vi "Database Driver Report Analysis.vi"(4 "Create Table":T4={"table"="", "column information"=[], "primary key (-1)"=-1, "use file? (F)"=FALSE}, 5 "Insert Data":T1, 6 "Options":T6=enum."Select Data", 7 "SQLTableData":T5, 8 "error in":errorcluster, 9 "SQL query":string, 10 "Select":enum16{"SelectWithQuery", "SelectWithColumn"}(ring), 11 "table":string) -> (0 "error out":errorcluster, 1 "tables":string[](array[string]), 2 "Database out":refnum<class "Database.lvclass">, 3 "data":string[][](array[string]))   [LabVIEW 2023, in "HardwareAbstractionLayer_LVOOP.lvlib" / "Database.lvclass"]
doc: "This VI used to Database action engine.\n\n// Defeault Case Select Query"
uses:
  Database.lvclass
  Control/DB Options.ctl
  <vilib>/addons/database/Auxilliary.llb/DB Tools Column Info.ctl
  <vilib>/addons/database/Auxilliary.llb/DB Tools DataTypes.ctl
  Control/DB Selection.ctl
  MYSQL Database_class/MYSQL Database.lvclass
  SQLite Database_class/SQLite Database.lvclass
  Database.lvclass/Database.ctl
  D:/eDCU LTT/VT LTT Project/Source Code/HardwareAbstractionLayer_LVOOP/Database/Database.lvclass
  D:/eDCU LTT/VT LTT Project/Source Code/HardwareAbstractionLayer_LVOOP/Database/MYSQL Database_class/MYSQL Database.lvclass
  D:/eDCU LTT/VT LTT Project/Source Code/HardwareAbstractionLayer_LVOOP/Database/SQLite Database_class/SQLite Database.lvclass
  <vilib>/addons/database/NI_Database_API.lvlib
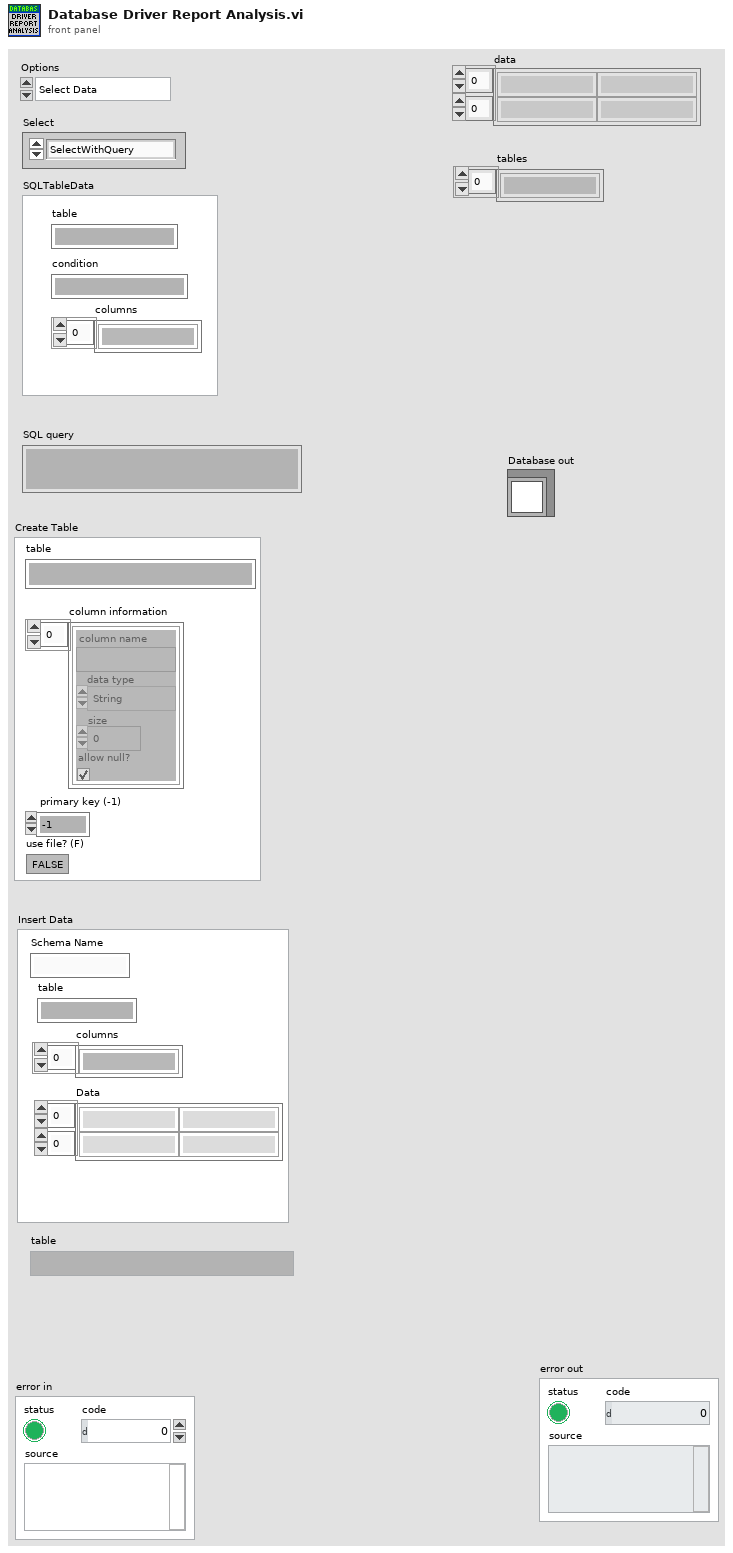
[diagram p1: front panel]
types:
  T1 = cluster{"table":string, "columns":string[], "Data":string[][], "Schema Name":string}
  T2 = typedef "NI_Database_API.lvlib/DB Tools Column Info.ctl" = cluster{"column name":string, "data type":T3, "size":i32, "allow null?":bool}
  T3 = typedef "NI_Database_API.lvlib/DB Tools DataTypes.ctl" = enum16{"String", "Long (I32)", "Single (SGL)", "Double (DBL)", "Date/Time", "Binary"}
  T4 = cluster{"table":string, "column information":T2[], "primary key (-1)":i32, "use file? (F)":bool}
  T5 = cluster{"table":string, "condition":string, "columns":string[]}
  T6 = typedef "HardwareAbstractionLayer_LVOOP.lvlib/Database.lvclass/DB Options.ctl" = enum16{"Init", "Select Data", "Insert Data", "Update Data", "Delete Data", "Execute Query", "Create Schema", "Create Table", "List Tables", "List Columns", "Close"}
  T7 = cluster{"DataSource Name":string, "userID":string, "password":string}
  T8 = enum16{"open", "replace", "create", "open or create", "replace or create", "replace or create with confirmation"}
  T9 = typedef "HardwareAbstractionLayer_LVOOP.lvlib/Database.lvclass/DB Selection.ctl" = string
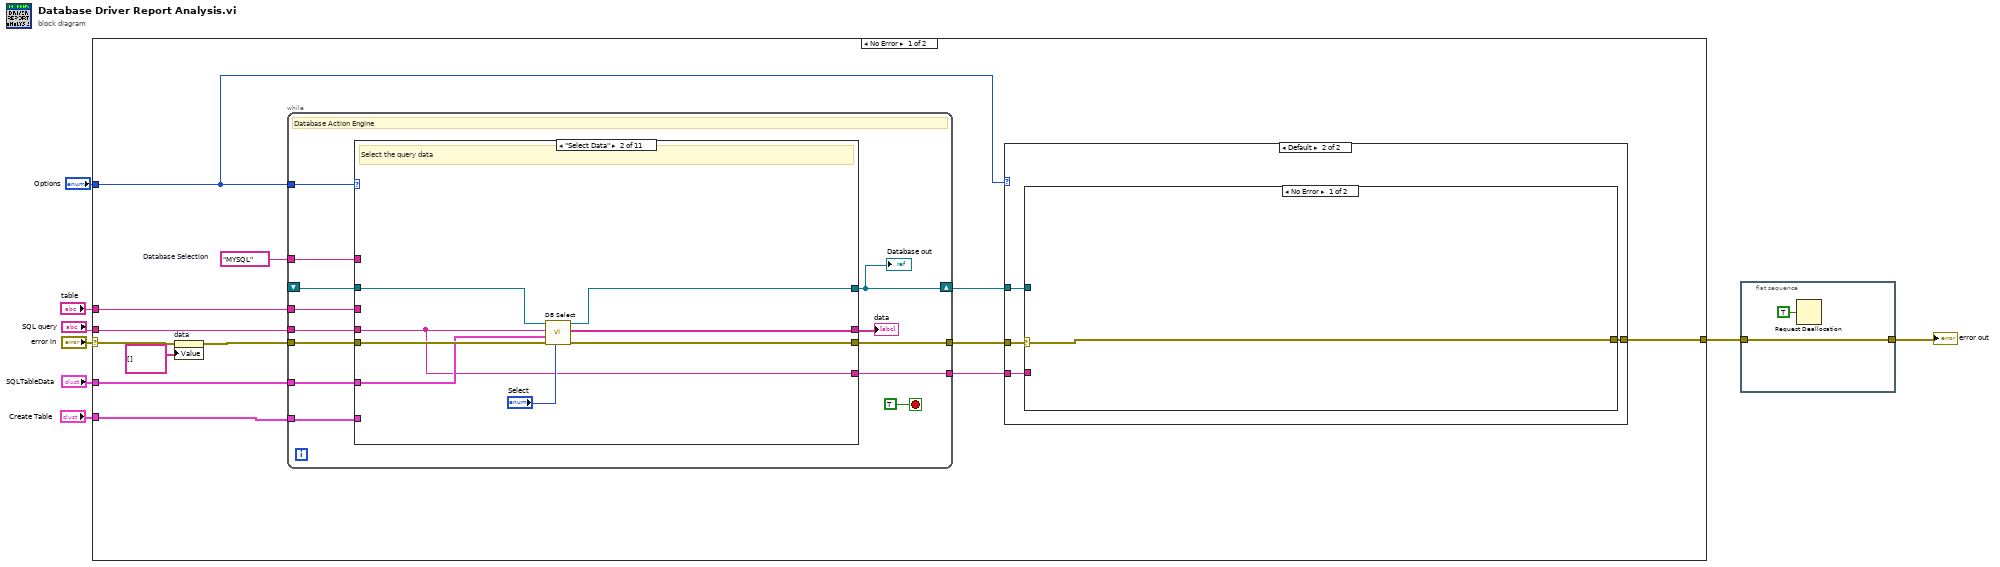
[diagram p0: block diagram]
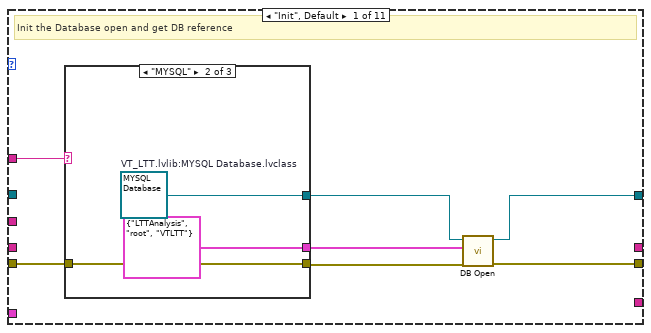
[diagram p2: hidden frame]
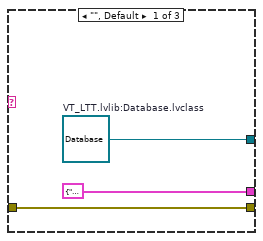
[diagram p3: hidden frame]
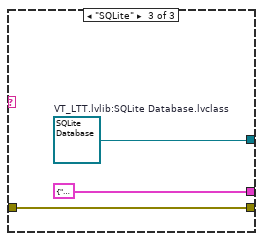
[diagram p4: hidden frame]
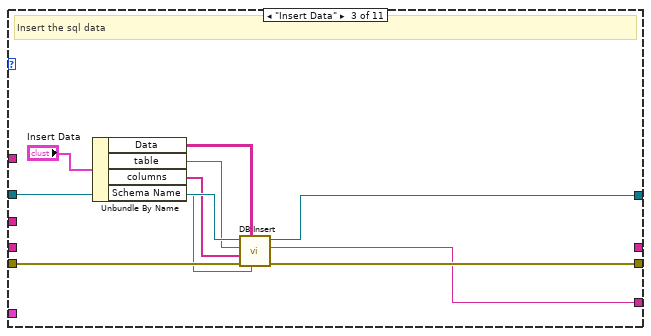
[diagram p5: hidden frame]
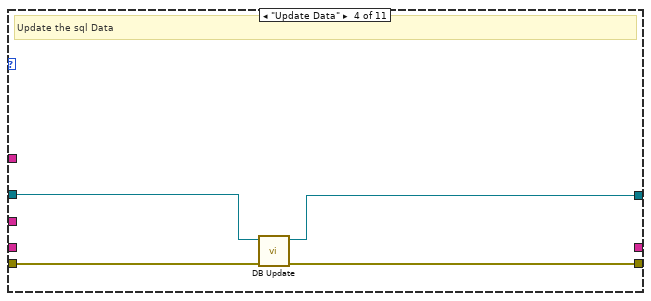
[diagram p6: hidden frame]
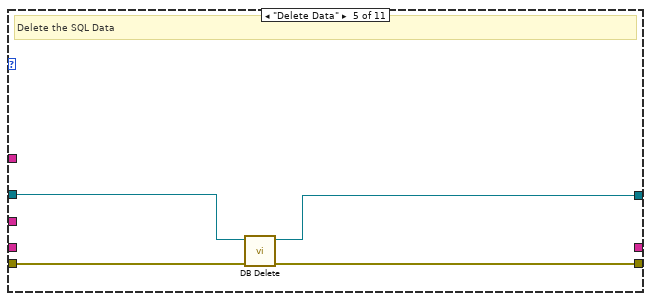
[diagram p7: hidden frame]
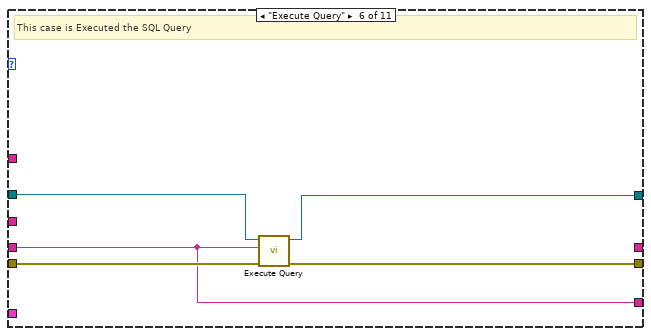
[diagram p8: hidden frame]
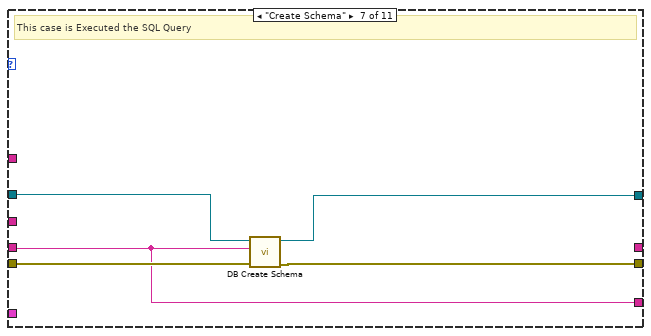
[diagram p9: hidden frame]
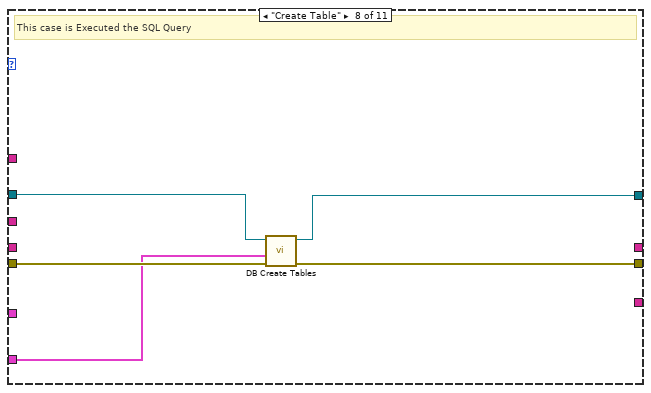
[diagram p10: hidden frame]
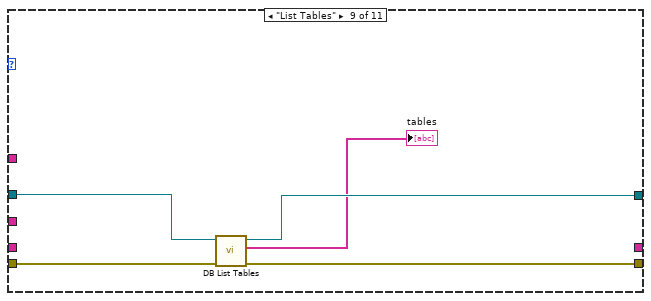
[diagram p11: hidden frame]
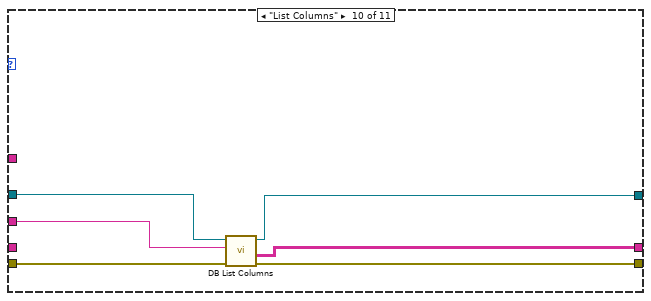
[diagram p12: hidden frame]
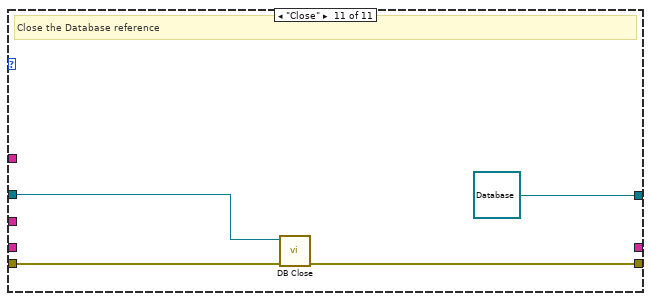
[diagram p13: hidden frame]
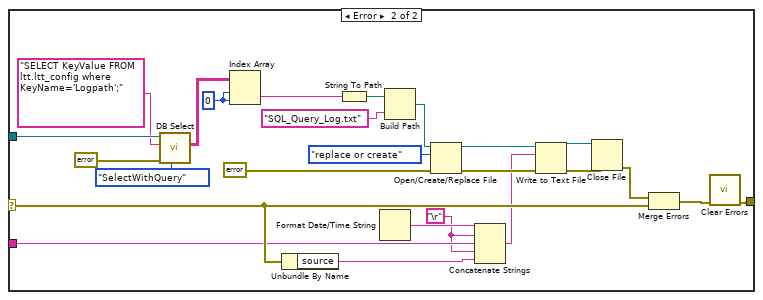
[diagram p15: hidden frame]
diagram:
  n1 = case shown="No Error" "error in" {
    selector: "error in" -> [w11 w138]
    tunnel: "SQL query" -> [w20 _]
    tunnel: "SQLTableData" -> [w19 _]
    tunnel: "Create Table" -> [w18 _]
    tunnel: "table" -> [w17 _]
    tunnel: [w14 w138] -> w2
    tunnel: "Options" -> [w13 _]
    frame No Error {
      w21 = T9 "MYSQL"  # Database Selection
      n2 = property on="data" class="Arr (strict)"(error in=w11, "Value"=string[][] [] ("data")) -> (error out=w10:errorcluster)  [unwired: 1 in, 1 out]
      n3 = while {
        tunnel: w13 -> [w33]
        tunnel: w21 -> [w32]
        shift-right: [w24] -> w12
        shift-left: _ -> [w29]
        tunnel: w20 -> [w28]
        tunnel: w19 -> [w27]
        tunnel: w18 -> [w25]
        tunnel: w17 -> [w23]
        tunnel: [w22] -> w15
        tunnel: w10 -> [w31]
        tunnel: [w30] -> w16
        stop <- TRUE stop-if-true
        # "Database Action Engine"
        n4 = case shown="\"Select Data\"" w33 {
          tunnel: w32 -> [w41 _ _ _ _ _ _ _ _ _ _]
          tunnel: w31 -> [w40 w58 w67 w72 w76 w81 w85 w89 w95 w101 w106]
          tunnel: [w35 w57 w66 w71 w75 w80 w84 w88 w94 w99 w105] -> w30
          tunnel: [w36 w55 w65 w69 w73 w78 w83 w90 w93 w100 refnum<class "Database.lvclass"> refnum ("Database out")] -> w24
          tunnel: w29 -> [_ w56 w68 w70 w74 w79 w86 w91 w96 w102 w104]
          tunnel: w28 -> [_ w51 _ _ _ w77 w82 _ _ _ _]
          tunnel: w27 -> [_ w53 _ _ _ _ _ _ _ _ _]
          tunnel: [_ w52 _ _ _ _ _ _ _ w97 _] -> w26
          tunnel: w25 -> [_ _ _ _ _ _ _ w87 _ _ _]
          tunnel: w23 -> [_ _ _ _ _ _ _ _ _ w98 _]
          tunnel: [_ w51 w59 _ _ w77 w82 _ _ _ _] -> w22
          frame "Init", Default {
            # "Init the Database open and get DB reference"
            n5 = case shown="\"MYSQL\"" w41 {
              tunnel: w40 -> [w44 w47 w50]
              tunnel: [w44 w47 w50] -> w39
              tunnel: [w43 w46 w49] -> w38
              tunnel: [T7 {"DataSource Name"="", "userID"="", "password"=""} ("DB") T7 {"DataSource Name"="LTTAnalysis", "userID"="root", "password"="VTLTT"} ("DB") T7 {"DataSource Name"="", "userID"="", "password"=""} ("DB")] -> w37
              frame "", Default {
                w43 = refnum<class "Database.lvclass"> refnum  # VT_LTT.lvlib:Database.lvclass
              }
              frame "MYSQL" {
                w46 = refnum<class "MYSQL Database.lvclass"> refnum  # VT_LTT.lvlib:MYSQL Database.lvclass
              }
              frame "SQLite" {
                w49 = refnum<class "SQLite Database.lvclass"> refnum  # VT_LTT.lvlib:SQLite Database.lvclass
              }
            }
            n6 = call-dynamic "DB Open.vi"("error in"=w39, "DB"=w37, "Database in"=w38) -> ("error out"=w35:errorcluster, "Database out"=w36:refnum<class "Database.lvclass">)  [unwired: 7 in]
          }
          frame "Select Data" {
            # "Select the query data"
            n7 = call-dynamic "DB Select.vi"("Select"="Select", "error in (no error)"=w58, "SQLTableData"=w53, "SQL query"=w51, "Database in"=w56) -> ("error out"=w57:errorcluster, "data"=w52:string[][], "Database out"=w55:refnum<class "Database.lvclass">)  [unwired: 4 in]
          }
          frame "Insert Data" {
            # "Insert the sql data"
            n8 = Unbundle By Name("Insert Data") -> ("Data"=w61:string[][], "table"=w63:string, "columns"=w62:string[], "Schema Name"=w60:string)
            n9 = call-dynamic "DB Insert.vi"("Schema Name"=w60, "Data"=w61, "error in (no error)"=w67, "columns"=w62, "table"=w63, "Database in"=w68) -> ("error out"=w66:errorcluster, "SQL"=w59:string, "Database out"=w65:refnum<class "Database.lvclass">)  [unwired: 3 in]
          }
          frame "Update Data" {
            # "Update the sql Data"
            n10 = call-dynamic "DB Update.vi"("error in (no error)"=w72, "Database in"=w70) -> ("error out"=w71:errorcluster, "Database out"=w69:refnum<class "Database.lvclass">)  [unwired: 8 in]
          }
          frame "Delete Data" {
            # "Delete the SQL Data"
            n11 = call-dynamic "DB Delete.vi"("error in (no error)"=w76, "Database in"=w74) -> ("error out"=w75:errorcluster, "Database out"=w73:refnum<class "Database.lvclass">)  [unwired: 8 in]
          }
          frame "Execute Query" {
            # "This case is Executed the SQL Query"
            n12 = call-dynamic "Execute Query.vi"("error in (no error)"=w81, "SQL query"=w77, "Database in"=w79) -> ("error out"=w80:errorcluster, "Database out"=w78:refnum<class "Database.lvclass">)  [unwired: 7 in]
          }
          frame "Create Schema" {
            # "This case is Executed the SQL Query"
            n13 = call-dynamic "DB Create Schema.vi"("error in (no error)"=w85, "SQL query"=w82, "Database in"=w86) -> ("error out"=w84:errorcluster, "Database out"=w83:refnum<class "Database.lvclass">)  [unwired: 7 in]
          }
          frame "Create Table" {
            # "This case is Executed the SQL Query"
            n14 = call-dynamic "DB Create Tables.vi"("error in (no error)"=w89, "Create Table"=w87, "Database in"=w91) -> ("error out"=w88:errorcluster, "Database out"=w90:refnum<class "Database.lvclass">)  [unwired: 7 in]
          }
          frame "List Tables" {
            n15 = call-dynamic "DB List Tables.vi"("error in (no error)"=w95, "Database in"=w96) -> ("error out"=w94:errorcluster, "tables"=→"tables":string[], "Database out"=w93:refnum<class "Database.lvclass">)  [unwired: 7 in]
          }
          frame "List Columns" {
            n16 = call-dynamic "DB List Columns.vi"("error in (no error)"=w101, "table"=w98, "Database in"=w102) -> ("error out"=w99:errorcluster, "tableDetails"=w97:string[][], "Database out"=w100:refnum<class "Database.lvclass">)  [unwired: 5 in, 1 out]
          }
          frame "Close" {
            # "Close the Database reference"
            n17 = call-dynamic "DB Close.vi"("error in"=w106, "Database in"=w104) -> ("error out"=w105:errorcluster)  [unwired: 8 in, 1 out]
          }
        }
        "data" <- w26
        "Database out" <- w24
      }
      n18 = case shown="Default" w13 {
        tunnel: w16 -> [w107 w111]
        tunnel: w15 -> [_ w110]
        tunnel: [w107 w109] -> w14
        tunnel: w12 -> [_ w108]
        frame "Init", "Close" {
        }
        frame Default {
          n19 = case shown="No Error" w111 {
            selector: w111 -> [w112 w120]
            tunnel: w110 -> [_ w117]
            tunnel: [w112 w113] -> w109
            tunnel: w108 -> [_ w129]
            frame No Error {
            }
            frame Error {
              w116 = "\r"
              w125 = 0 ("disabled index (col)")
              n20 = call-dynamic "DB Select.vi"("Select"=enum16{"SelectWithQuery", "SelectWithColumn"}."SelectWithQuery", "error in (no error)"=errorcluster {"status"=FALSE, "code"=0, "source"=""}, "SQL query"="SELECT KeyValue FROM ltt.ltt_config where KeyName='Logpath';", "Database in"=w129) -> ("data"=w126:string[][])  [unwired: 5 in, 2 out]
              n21 = Index Array(array=w126, index (row)=w125, index (col)=w125) -> (element=w124:string)
              n22 = Unbundle By Name(w120) -> ("source"=w115:string)
              n23 = String To Path(string=w124) -> (path=w123:path)
              n24 = Format Date/Time String() -> (date/time string=w119:string)  [unwired: 3 in]
              n25 = Build Path(base path=w123, name or relative path="SQL_Query_Log.txt") -> (appended path=w131:path)
              n26 = Open/Create/Replace File(file path (use dialog)=w131, error in=errorcluster {"status"=FALSE, "code"=0, "source"=""}, operation (0:open)=T8."replace or create") -> (refnum out=w135:refnum<file>, error out=w134:errorcluster)  [unwired: 3 in, 1 out]
              n27 = Concatenate Strings(w119, w116, w117, w116, w115) -> (w118:string)
              n28 = Write to Text File(file (use dialog)=w135, text=w118, error in=w134) -> (refnum out=w137:refnum<file>, error out=w136:errorcluster)  [unwired: 1 in, 1 out]
              n29 = Close File(refnum=w137, error in=w136) -> (error out=w130:errorcluster)  [unwired: 1 out]
              n30 = Merge Errors(w130, w120) -> (w114:errorcluster)
              n31 = call <vilib>:"Clear Errors.vi"("error in (no error)"=w114) -> ("error out"=w113:errorcluster)  [unwired: 5 in, 1 out]
            }
          }
        }
      }
    }
    frame Error {
    }
  }
  n32 = flat-sequence {
    tunnel: w2 -> [w140]
    tunnel: [w140] -> w1
    frame #0 {
      n33 = Request Deallocation(TRUE ("flag")) -> ()
    }
  }
  "error out" <- w1
